vi "Check Status.vi"(8 "Error In":errorcluster, 10 "Status":i32, 11 "labssh2 Shared Library In":path=path "") -> (0 "Error Out":errorcluster, 3 "labssh2 Shared Library Out":path)   [LabVIEW 2017, in "Toolkit.lvlib"]
uses:
  Toolkit.lvlib
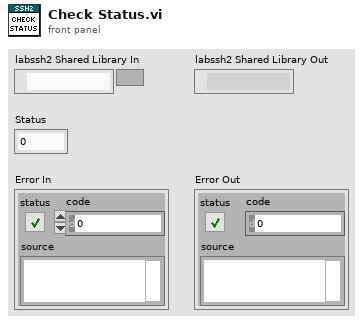
[diagram p1: front panel]
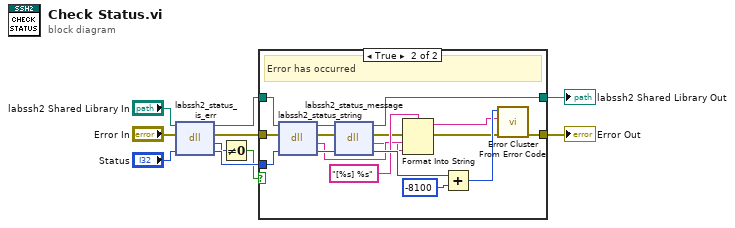
[diagram p0: block diagram]
diagram:
  n1 = dll-call lib="D:/Users/cfield/Code/Field R&D Services/SSH/LabSSH2/LabVIEW/trunk/src/LabSSH2/Private/labssh2.*" fn="labssh2_status_is_err"(path in="labssh2 Shared Library In", error in="Error In", "status"="Status") -> (path out=w9:path, error out=w7:errorcluster, "bool"=w4:i32, "status"=w5:i32)  [unwired: 1 in]
  n2 = Not Equal To 0?(x=w4) -> (x != 0?=w3:bool)
  n3 = case shown="True" w3 {
    tunnel: w9 -> [w12 w26]
    tunnel: w7 -> [w11 w25]
    tunnel: w5 -> [_ w24]
    tunnel: [w12 w23] -> w2
    tunnel: [w11 w20] -> w1
    frame False {
      # "No error"
    }
    frame True {
      # "Error has occurred"
      n4 = dll-call lib="D:/Users/cfield/Code/Field R&D Services/SSH/LabSSH2/LabVIEW/trunk/src/LabSSH2/Private/labssh2.*" fn="labssh2_status_string"(path in=w26, error in=w25, "status"=w24) -> (path out=w27:path, error out=w28:errorcluster, "string"=w14:string, "status"=w29:i32)  [unwired: 1 in]
      n5 = dll-call lib="D:/Users/cfield/Code/Field R&D Services/SSH/LabSSH2/LabVIEW/trunk/src/LabSSH2/Private/labssh2.*" fn="labssh2_status_message"(path in=w27, error in=w28, "status"=w29) -> (path out=w23:path, error out=w17:errorcluster, "message"=w13:string, "status"=w22:i32)  [unwired: 1 in]
      n6 = Format Into String(format string="[%s] %s", error in=w17, w14, w13) -> (resulting string=w15:string, error out=w16:errorcluster)  [unwired: 1 in]
      n7 = Add(x=w22, y=-8100) -> (x+y=w19:i32)
      n8 = call <vilib>:"Error Cluster From Error Code.vi"("error in (no error)"=w16, "error message (\"\")"=w15, "error code (0)"=w19) -> ("error out"=w20:errorcluster)  [unwired: 6 in]
    }
  }
  "labssh2 Shared Library Out" <- w2
  "Error Out" <- w1
